vi "Save_plot_routine.vi"(2 "Show Smooth":bool, 3 "First Plot data":cluster{"Xo":dbl, "Delta X":dbl, dbl[]}[](array[cluster]) {"?" format="%.2f"; "Delta X" format="%.2f"; "Xo" format="%.2f"}, 4 "Second Plot data":cluster{"Xo":dbl, "Delta X":dbl, dbl[]}[](array[cluster]) {"?" format="%.2f"; "Delta X" format="%.2f"; "Xo" format="%.2f"}) -> ()   [LabVIEW 2010]
uses:
  Controls/Post_Process.ctl
  Globals/Meas_global.vi
  Globals/Constants_global.vi
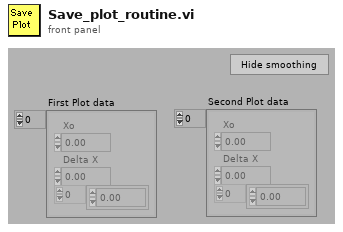
[diagram p1: front panel]
types:
  T1 = typedef "Post_Process.ctl" = enum16{"Take New Data", "Post Process Raw Data File"}
  T2 = cluster{"Name":string, "X":dbl, "Y":dbl, "Z":dbl}[]
  T3 = typedef "Graph_Type.ctl" = enum16{"Show no graph", "Voltage trace", "Velocity trace", "Vel histogram", "Spectrum", "f.E(f) v Log f", "Auto-Corr"}
  T4 = cluster{"Plot 1":u16, "Plot 2":u16, "Save graph":u16, "Plot Type":T3}
  T5 = cluster{"Start Index":i32, "End Index":i32, "Smoothing":enum16{"Linear", "Logarithmic"}, "Number of smoothed estimates":i32, "X axis":cluster{"Mapping":u16, "Format":u16}, "Y axis":cluster{"Mapping":u16, "Format":u16}, "Use Whole Input Array?":bool}[]
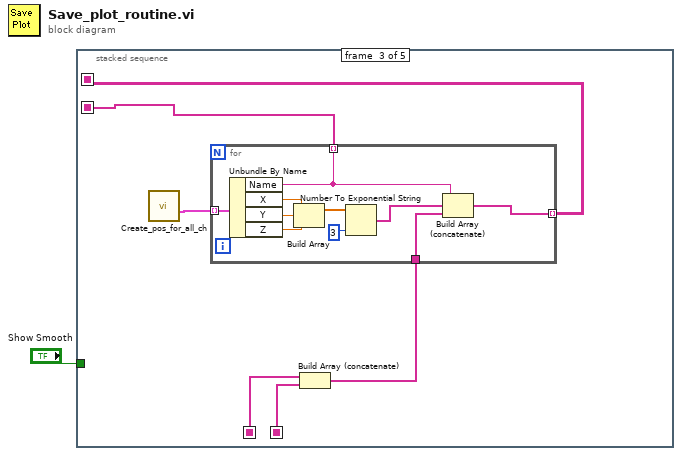
[diagram p0: block diagram]
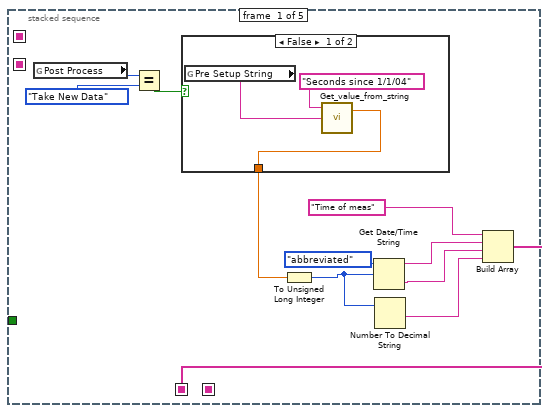
[diagram p2: hidden frame]
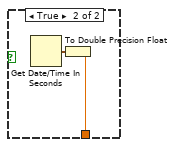
[diagram p3: hidden frame]
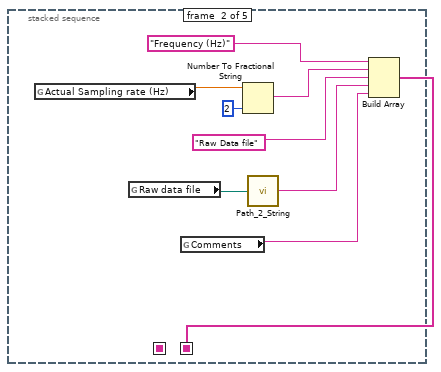
[diagram p4: hidden frame]
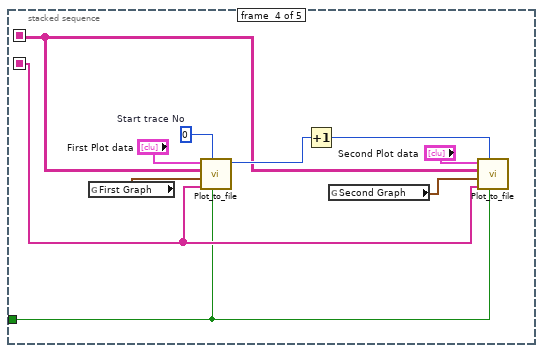
[diagram p5: hidden frame]
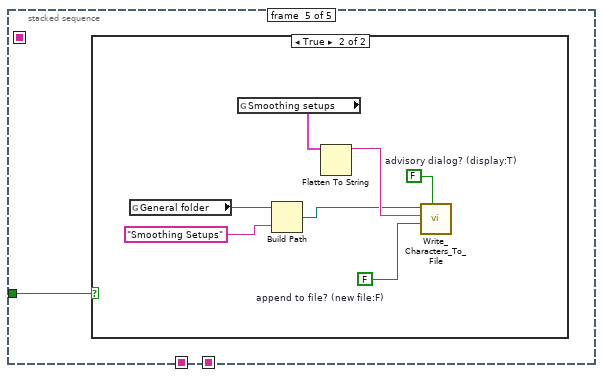
[diagram p6: hidden frame]
diagram:
  n1 = stacked-sequence {
    seq-local: [_ _ w32 _ _] -> [_ _ _ w46 _]
    seq-local: [_ _ w27 _ _] -> [_ _ _ w44 _]
    seq-local: [w5 _ _ _ _] -> [_ _ w30 _ _]
    seq-local: [_ w22 _ _ _] -> [_ _ w29 _ _]
    tunnel: "Show Smooth" -> [_ _ _ w43 w53]
    frame #0 {
      n2 = global read "Meas_global.vi" "Post Process"() -> (w11:T1)
      n3 = Equal?(x=w11, y=Post_Process."Take New Data" ("Post Process")) -> (x = y?=w10:bool)
      n4 = case shown="False" w10 {
        tunnel: [w13 w17] -> w9
        frame False {
          n5 = global read "Meas_global.vi" "Pre Setup String"() -> (w14:string)
          n6 = call "Get_value_from_string.vi"("Input string"=w14, "Variable name"="Seconds since 1/1/04") -> ("Value"=w13:dbl)  [unwired: 1 in, 1 out]
        }
        frame True {
          n7 = Get Date/Time In Seconds() -> (seconds since 1Jan1904=w16:timestamp)
          n8 = To Double Precision Float(number=w16) -> (double precision float=w17:dbl)
        }
      }
      n9 = To Unsigned Long Integer(number=w9) -> (unsigned 32bit integer=w4:u32)
      n10 = Get Date/Time String(date format (0)=enum16{"short", "long", "abbreviated"}."abbreviated", seconds (now)=w4) -> (date string=w7:string, time string=w6:string)  [unwired: 1 out]
      n11 = Number To Decimal String(number=w4) -> (decimal integer string=w3:string)  [unwired: 1 out]
      n12 = Build Array("Time of meas", w7, w6, w3) -> (w5:string[])
    }
    frame #1 {
      n13 = global read "Meas_global.vi" "Actual Sampling rate (Hz)"() -> (w26:dbl)
      n14 = global read "Meas_global.vi" "Raw data file"() -> (w19:path)
      n15 = global read "Meas_global.vi" "Comments"() -> (w20:string)
      n16 = Number To Fractional String(number=w26, precision (6)=i16 2) -> (F-format string=w23:string)  [unwired: 2 out]
      n17 = call "Path_2_String.vi"("Real Path"=w19) -> ("Path String"=w18:string)
      n18 = Build Array("Frequency (Hz)", w23, "Raw Data file", w18, w20) -> (w22:string[])
    }
    frame #2 {
      n19 = call "Create_pos_for_all_ch.vi"() -> ("Positions for all Ch"=w31:T2)  [unwired: 6 out]
      n20 = Build Array (concatenate)(w30, w29) -> (w28:string[])
      n21 = for {
        tunnel: w31 -> [w42] mode=indexing
        tunnel: w28 -> [w34]
        tunnel: [w35] -> w32 mode=indexing
        tunnel: [w33] -> w27 mode=indexing
        n22 = Unbundle By Name(w42) -> ("Name"=w33:string, "X"=w41:dbl, "Y"=w40:dbl, "Z"=w39:dbl)
        n23 = Build Array(w41, w40, w39) -> (w37:dbl[])
        n24 = Number To Exponential String(number=w37, precision (6)=3) -> (E-format string=w36:string[])  [unwired: 2 out]
        n25 = Build Array (concatenate)(w33, w36, w34) -> (w35:string[])
      }
    }
    frame #3 {
      w50 = 0  # Start trace No
      n26 = global read "Meas_global.vi" "First Graph"() -> (w51:T4)
      n27 = call "Plot_to_file.vi"("Show Smooth"=w43, "Start trace No"=w50, "Trace names"=w44, "Graph"=w51, "Plot file label"=w46, "Plot data"="First Plot data") -> ("End trace No"=w49:i32)  [unwired: 5 out]
      n28 = Increment(x=w49) -> (x+1=w48:i32)
      n29 = global read "Meas_global.vi" "Second Graph"() -> (w45:T4)
      n30 = call "Plot_to_file.vi"("Show Smooth"=w43, "Start trace No"=w48, "Trace names"=w44, "Graph"=w45, "Plot file label"=w46, "Plot data"="Second Plot data") -> ()  [unwired: 6 out]
    }
    frame #4 {
      n31 = case shown="True" w53 {
        frame False {
        }
        frame True {
          w57 = FALSE  # advisory dialog? (display:T)
          w58 = FALSE  # append to file? (new file:F)
          n32 = global read "Constants_global.vi" "General folder"() -> (w56:path)
          n33 = global read "Meas_global.vi" "Smoothing setups"() -> (w60:T5)
          n34 = Build Path(base path=w56, name or relative path="Smoothing Setups" ("Substring")) -> (appended path=w54:path)
          n35 = Flatten To String(anything=w60) -> (data string=w59:string)  [unwired: 1 in, 4 out]
          n36 = call "Write_Characters_To_File.vi"("file path (dialog if empty)"=w54, "advisory dialog? (display:T)"=w57, "character string"=w59, "append to file? (new file:F)"=w58) -> ()  [unwired: 1 in, 4 out]
        }
      }
    }
  }
